vi "Manage Background Music.vi"(8 "error in (no error)":errorcluster, 9 "Music Paused":bool, 10 "Dyn Sounds Path":path, 11 "Sounds":T1[](array[typedef]) {"Task ID" format="%.0x"}) -> (0 "error out":errorcluster, 3 "Sounds Out":T1[](array[typedef]) {"Task ID" format="%.0x"}, 5 "BackGround Track":string)   [LabVIEW 2021, in "Sound Manager.lvlib"]
uses:
  Sound Manager.lvlib
  Typedefs/Sound Data.ctl
  Typedefs/Sound Effects.ctl
  <vilib>/sound2/lvsound2.llb/Sound Output Task ID.ctl
  <vilib>/numeric/Random Number (Range) DBL.vi
  <vilib>/sound2/lvsound2.llb/Sound Output Set Volume (Single).vi
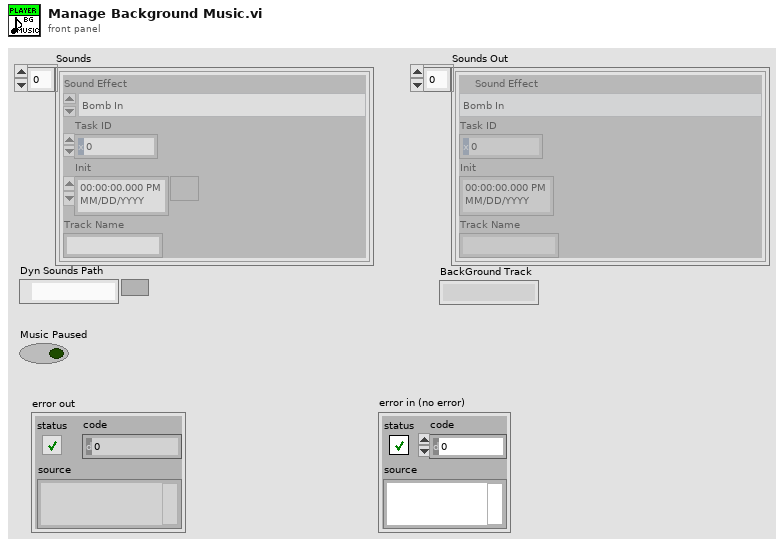
[diagram p1: front panel]
types:
  T1 = typedef "Sound Manager.lvlib/Sound Data.ctl" = cluster{"Sound Effect":T2, "Task ID":T3, "Init":timestamp, "Track Name":string}
  T2 = typedef "Sound Manager.lvlib/Sound Effects.ctl" = enum16{"Bomb In", "Bomb Out", "Bomb Touched", "Game Over", "Victory", "Eat", "10 Fruits", "Eat2", "Eat3", "Eat4", "MaxShield", "Shield", "10p", "Grape In", "Grape Out", "20p", "30p", "40p", "50p", "60p", "70p", "80p", "90p", "100p", "All shields cracked", "Mouse In", "Mouse Out", "Mouse Eaten", "Grape Eaten", "States Recover", "Broken Shield", "Bonus", "Happy Time", "explode", "Game over musica", "Back Music", "Shield Catch", "Evil lough", "Cricket In", "Cricket eaten", "Lets Go", "Jump1", "Jump2", "Jump3", "Unstoppable", "Troll Music", "winner", "menu"}
  T3 = typedef "Sound Output Task ID.ctl" = u32
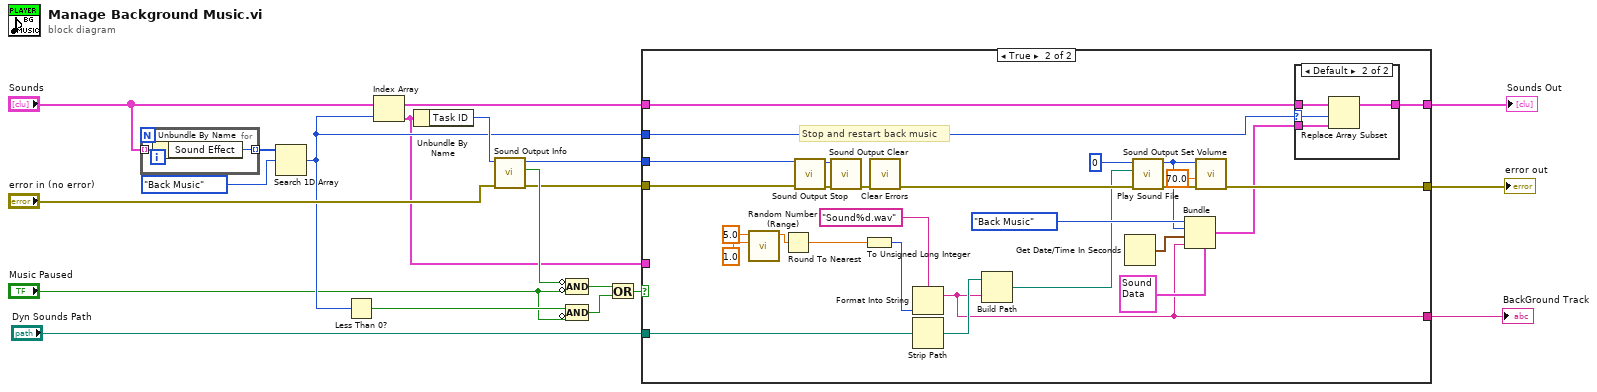
[diagram p0: block diagram]
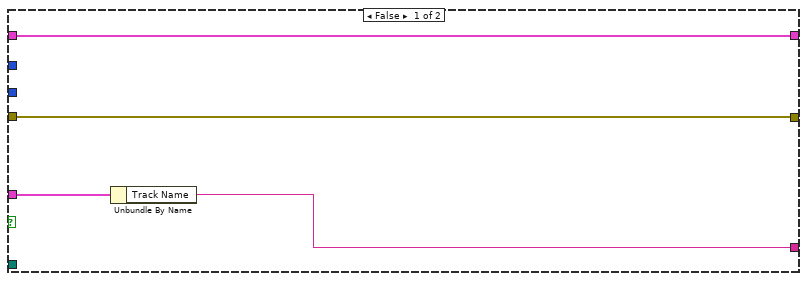
[diagram p2: hidden frame]
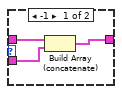
[diagram p3: hidden frame]
diagram:
  n1 = for {
    tunnel: "Sounds" -> [w21] mode=indexing
    tunnel: [w20] -> w17 mode=indexing
    n2 = Unbundle By Name(w21) -> ("Sound Effect"=w20:T2)
  }
  n3 = Search 1D Array(1D array=w17, element=Sound_Effects."Back Music") -> (index of element=w8:i32)  [unwired: 1 in]
  n4 = Less Than 0?(x=w8) -> (x < 0?=w7:bool)
  n5 = Index Array(array="Sounds", index=w8) -> (element=w2:T1)
  n6 = Unbundle By Name(w2) -> ("Task ID"=w19:T3)
  n7 = call <vilib>:"Sound Output Info.vi"("error in (no error)"="error in (no error)", "task ID"=w19) -> ("error out"=w12:errorcluster, "is playing?"=w15:bool, "task ID out"=w13:T3)  [unwired: 6 in, 1 out]
  n8 = Compound Arithmetic op=AND(invert w15, invert "Music Paused") -> (w14:bool)
  n9 = Compound Arithmetic op=AND(w7, invert "Music Paused") -> (w4:bool)
  n10 = Or(x=w14, y=w4) -> (x .or. y?=w5:bool)
  n11 = case shown="True" w5 {
    tunnel: w13 -> [_ w51]
    tunnel: w12 -> [w24 w50]
    tunnel: "Sounds" -> [w25 w48]
    tunnel: [w24 w42] -> w9
    tunnel: w8 -> [_ w40]
    tunnel: [w25 w39] -> w10
    tunnel: "Dyn Sounds Path" -> [_ w30]
    tunnel: w2 -> [w23 _]
    tunnel: [w22 w26] -> w1
    frame False {
      n12 = Unbundle By Name(w23) -> ("Track Name"=w22:string)
    }
    frame True {
      # "Stop and restart back music"
      n13 = call-poly <vilib>:"Random Number (Range).vi"("lower bound (0)"=1.0 ("Low"), "upper bound (100)"=5.0 ("High")) -> ("number"=w36:dbl)  [unwired: 9 in]
      n14 = Round To Nearest(number=w36) -> (nearest integer value=w35:dbl)
      n15 = call <vilib>:"Sound Output Stop.vi"("error in (no error)"=w50, "task ID"=w51) -> ("error out"=w49:errorcluster, "task ID out"=w52:T3)  [unwired: 8 in]
      n16 = call <vilib>:"Sound Output Clear.vi"("error in (no error)"=w49, "task ID"=w52) -> ("error out"=w53:errorcluster)  [unwired: 9 in]
      n17 = To Unsigned Long Integer(number=w35) -> (unsigned 32bit integer=w33:u32)
      n18 = call <vilib>:"Clear Errors.vi"("error in (no error)"=w53) -> ("error out"=w45:errorcluster)  [unwired: 5 in, 1 out]
      n19 = Format Into String(format string="Sound%d.wav", w33) -> (resulting string=w26:string)  [unwired: 2 in, 1 out]
      n20 = Strip Path(path=w30) -> (stripped path=w31:path)  [unwired: 1 out]
      n21 = Build Path(base path=w31, name or relative path=w26) -> (appended path=w32:path)
      n22 = Get Date/Time In Seconds() -> (seconds since 1Jan1904=w28:timestamp)
      n23 = call <vilib>:"Play Sound File.vi"("error in (no error)"=w45, "path"=w32, "device ID"=u32 0) -> ("error out"=w46:errorcluster, "task ID"=w43:T3)  [unwired: 7 in]
      n24 = Bundle(cluster=T1 {"Sound Effect"=enum."Bomb In", "Task ID"=0, "Init"=timestamp(0 s since 1904-01-01), "Track Name"=""} ("Cluster"), "Sound Effect"=Sound_Effects."Back Music" ("element"), "Task ID"=w43, "Init"=w28, "Track Name"=w26) -> (w41:T1)
      n25 = call-poly <vilib>:"Sound Output Set Volume.vi"("error in (no error)"=w46, "volume"=70.0, "task ID"=w43) -> ("error out"=w42:errorcluster)  [unwired: 7 in, 1 out]
      n26 = case shown="Default" w40 {
        selector: w40 -> [_ w58]
        tunnel: w48 -> [w56 w60]
        tunnel: w41 -> [w54 w59]
        tunnel: [w55 w57] -> w39
        frame -1 {
          n27 = Build Array (concatenate)(w56, w54) -> (w55:T1[])
        }
        frame Default {
          n28 = Replace Array Subset(array=w60, new element=w59, index=w58) -> (w57:T1[])
        }
      }
    }
  }
  "Sounds Out" <- w10
  "error out" <- w9
  "BackGround Track" <- w1
